vi "Place myDevice FPGA VI.vi"() -> ()   [LabVIEW 2017]
panel:
  in  "NI.myDevice.Enable Transmission":bool
  in  "NI.myDevice.Serial Settings":cluster{"slaveID":i16, "baud rate":i16}
  # "Controls that are intended to be exposed to the user SHOULD have your device name prepended so the input created by the FPGA Developer has the correct default name."
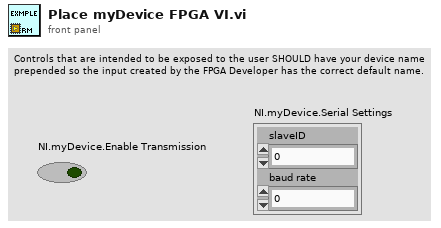
[diagram p1: front panel]
types:
  T1 = cluster{"SCLK":refnum<k21>, "MOSI":refnum<k21>, "MISO":refnum<k21>, "SS 0":refnum<k21>, "SS 1":refnum<k21>, "SS 2":refnum<k21>, "SS 3":refnum<k21>}
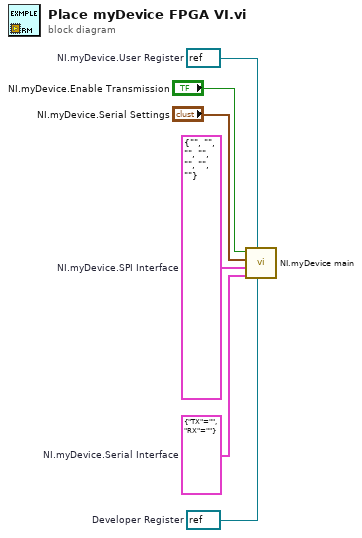
[diagram p0: block diagram]
diagram:
  w1 = refnum<k21> refnum  # Developer Register
  w2 = refnum<k21> refnum  # NI.myDevice.User Register
  w5 = cluster{"TX":refnum<k21>, "RX":refnum<k21>} {"TX"="", "RX"=""}  # NI.myDevice.Serial Interface
  w6 = T1 {"SCLK"="", "MOSI"="", "MISO"="", "SS 0"="", "SS 1"="", "SS 2"="", "SS 3"=""}  # NI.myDevice.SPI Interface
  n1 = call "NI.myDevice main.vi"("Developer Register"=w1, "NI.myDevice.User Register"=w2, "NI.myDevice.Serial Interface"=w5, "NI.myDevice.SPI Interface"=w6, "NI.myDevice.Serial Settings"="NI.myDevice.Serial Settings", "NI.myDevice.Enable Transmission"="NI.myDevice.Enable Transmission") -> ()  [unwired: 6 in]
